vi "Save_Info.vi"(8 "error in (no error)":errorcluster, 11 "AB_Application in":refnum<class "AB_Application.lvclass">) -> (0 "error out":errorcluster, 3 "AB_Application out":refnum<class "AB_Application.lvclass">)   [LabVIEW 2020, in "AB_Application.lvclass"]
uses:
  <vilib>/AppBuilder/AB_Classes/Application/AB_Application.lvclass
  e:/builds/penguin/labview/branches/2020/dev/dist/vi.lib/AppBuilder/AB_Classes/Build/AB_Build.lvclass
  <vilib>/AppBuilder/RW_Project/AB_RW_Project_App_Data.ctl
  <vilib>/AppBuilder/RW_Project/AB_RW_Project_App_EmbeddedServerConfiguration_Data.ctl
  <vilib>/AppBuilder/RW_Project/AB_RW_Project_PropBag_Action.ctl
  <vilib>/AppBuilder/AB_Classes/Application/AB_Application.lvclass/AB_Application.ctl
  <vilib>/AppBuilder/AB_Classes/TargetFile/AB_Targetfile.lvclass
  <vilib>/AppBuilder/AB_Classes/Build/AB_Build.lvclass
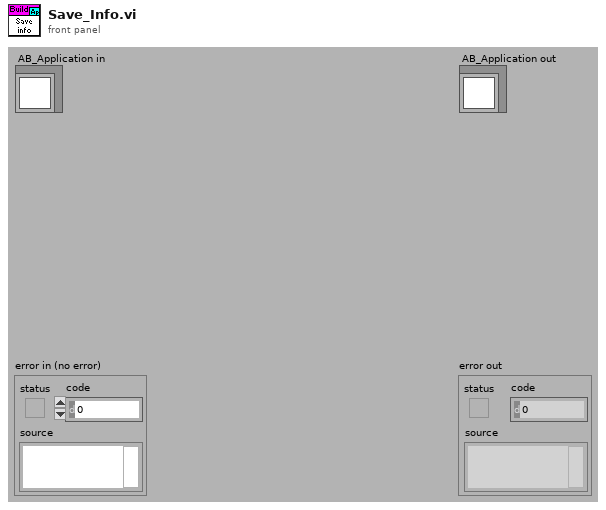
[diagram p1: front panel]
types:
  T1 = typedef "AB_RW_Project_App_Data.ctl" = cluster{"INI_itemID":string, "INI_GUID":string, "aliasItemID":string, "aliasGUID":string, "waitDebugging":bool, "copyErrors":bool, "useFFRTE":bool, "includeHWConfig":bool, "showHWConfig":bool, "winsec.certificate":string, "winsec.timestamp":string, "winsec.description":string, "winsec.manifestItemID":string, "web service itemIDs":string[], "Embedded Server Configuration":T2, "Server Type":enum32{"NI Web Server", "Application Web Server"}}
  T2 = typedef "AB_RW_Project_App_EmbeddedServerConfiguration_Data.ctl" = cluster{"HTTP enabled?":bool, "HTTP port":i32, "HTTPS enabled?":bool, "HTTPS port":i32, "SSL certificate file":path}
  T3 = typedef "AB_RW_Project_PropBag_Action.ctl" = enum16{"read", "write", "clear", "readPrevious", "writePrevious", "clearPrevious"}
  T4 = enum32{"NI Web Server", "Application Web Server"}
  T5 = typedef "AB_Build.ctl" = cluster{"buildSpecName":string, "buildSpecDescription":string, "destinations":refnum<class "AB_Destination.lvclass">[], "exclusionOption":T6, "defaultLanguage":string, "supportedLanguages":string[], "excludedDirectories":path[], "buildContext":refnum<vi>, "buildObject":T7, "preview":bool, "programatic":bool, "progressBarEvents":T8, "userLog_Path":path, "preActionID":string, "preAction_Path":path, "postActionID":string, "postAction_Path":path, "eng_checkForBrokenVIs?":bool, "eng_verboseLinkerErrors?":bool, "localDest_Path":path, "targetDest_Path":path, "removeVIObject":u16, "cache":refnum<class "PreviewCache.lvclass">, "use cache":bool, "previewCache_ID":string, "buildCache_ID":string, "eng_TempLocalDest_Path":path, "eng_collectDependencies?":bool, "versionInfo":cluster{"buildVersion":cluster{"major":u16, "minor":u16, "patch":u16, "build":u16}, "autoIncrement":bool}, "eng_enableVIChecksums":bool}
  T6 = typedef "AB_Exclusion_Option.ctl" = cluster{"typedefs":bool, "polymorphicVIs":bool, "unusedLibraryItems":bool, "modifyLibraryFile":bool, "edit-timeDependencies":bool, "inlineVIs":bool, "dependent PPLs":bool, "dependent DLLs":bool}
  T7 = typedef "ItemRef.ctl" = u64
  T8 = typedef "provcom_ProgressBar_Events.ctl" = cluster{"newJob":refnum<user-event>, "newItem":refnum<user-event>, "errorMsg":T9, "cancel":refnum<user-event>}
  T9 = typedef "mxLvBuildError.ctl" = refnum<user-event>
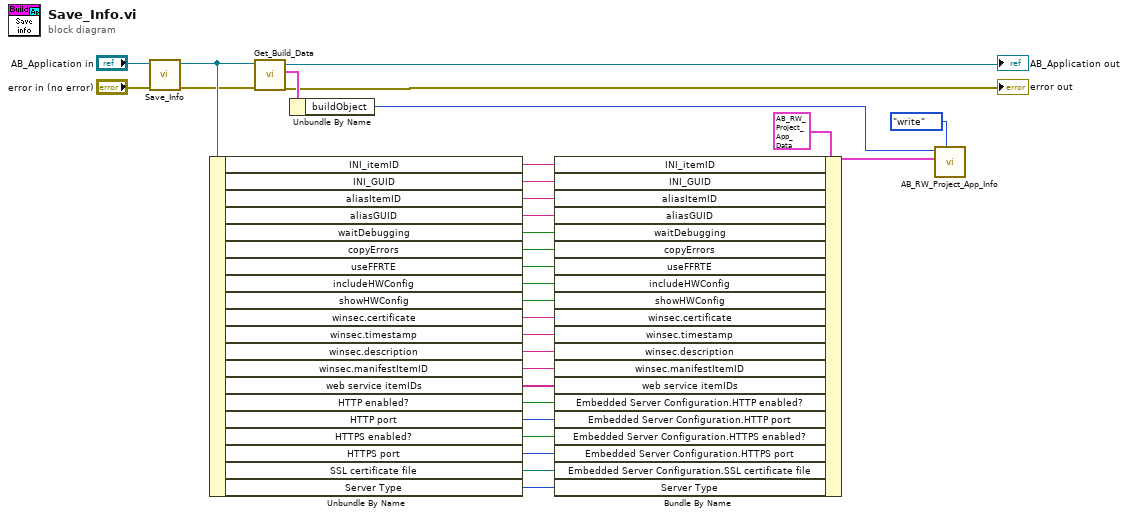
[diagram p0: block diagram]
diagram:
  n1 = call-parent "Save_Info.vi"("error in (no error)"="error in (no error)", "AB_Targetfile in"="AB_Application in") -> ("error out"=w17:errorcluster, "AB_Targetfile out"=w18:refnum<class "AB_Application.lvclass">)  [unwired: 8 out]
  n2 = Unbundle By Name(w18) -> ("INI_itemID"=w27:string, "INI_GUID"=w16:string, "aliasItemID"=w26:string, "aliasGUID"=w15:string, "waitDebugging"=w25:bool, "copyErrors"=w24:bool, "useFFRTE"=w23:bool, "includeHWConfig"=w22:bool, "showHWConfig"=w21:bool, "winsec.certificate"=w14:string, "winsec.timestamp"=w13:string, "winsec.description"=w12:string, "winsec.manifestItemID"=w11:string, "web service itemIDs"=w9:string[], "HTTP enabled?"=w8:bool, "HTTP port"=w7:i32, "HTTPS enabled?"=w6:bool, "HTTPS port"=w5:i32, "SSL certificate file"=w4:path, "Server Type"=w1:T4)
  n3 = call <vilib>:"Get_Build_Data.vi"("error in (no error)"=w17, "Class in"=w18) -> ("error out"=→"error out":errorcluster, "data"=w19:T5, "Class out"=→"AB_Application out":refnum<class "AB_Application.lvclass">)  [unwired: 7 out]
  n4 = Unbundle By Name(w19) -> ("buildObject"=w10:T7)
  n5 = Bundle By Name(cluster=T1 {"INI_itemID"="", "INI_GUID"="", "aliasItemID"="", "aliasGUID"="", "waitDebugging"=FALSE, "copyErrors"=FALSE, "useFFRTE"=FALSE, "includeHWConfig"=FALSE, "showHWConfig"=FALSE, "winsec.certificate"="", "winsec.timestamp"="", "winsec.description"="", "winsec.manifestItemID"="", "web service itemIDs"=[], "Embedded Server Configuration"={"HTTP enabled?"=FALSE, "HTTP port"=0, "HTTPS enabled?"=FALSE, "HTTPS port"=0, "SSL certificate file"=path ""}, "Server Type"=enum."NI Web Server"} ("applicationInfo in"), "INI_itemID"=w27, "INI_GUID"=w16, "aliasItemID"=w26, "aliasGUID"=w15, "waitDebugging"=w25, "copyErrors"=w24, "useFFRTE"=w23, "includeHWConfig"=w22, "showHWConfig"=w21, "winsec.certificate"=w14, "winsec.timestamp"=w13, "winsec.description"=w12, "winsec.manifestItemID"=w11, "web service itemIDs"=w9, "Embedded Server Configuration.HTTP enabled?"=w8, "Embedded Server Configuration.HTTP port"=w7, "Embedded Server Configuration.HTTPS enabled?"=w6, "Embedded Server Configuration.HTTPS port"=w5, "Embedded Server Configuration.SSL certificate file"=w4, "Server Type"=w1) -> (w20:T1)
  n6 = call <vilib>:"AB_RW_Project_App_Info.vi"("action"=AB_RW_Project_PropBag_Action."write", "applicationInfo in"=w20, "Object In"=w10) -> ()  [unwired: 2 in, 7 out]
